vi "remove.issue.from.submap.vi"(10 "issue id":i32, 11 "map in":T1) -> (3 "map out":T1)   [LabVIEW 2024, in "manager_daemon.lvclass"]
uses:
  manager_daemon.lvclass
  type_defs/sub-map--map.ctl
  type_defs/SubData--cluster.ctl
  manager_daemon.lvclass/manager_daemon.ctl
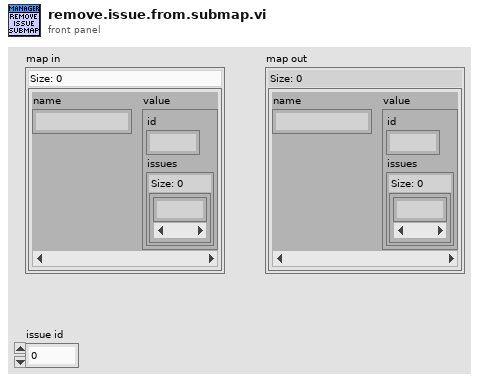
[diagram p1: front panel]
types:
  T1 = typedef "manager_daemon.lvclass/sub-map--map.ctl" = map{string, T2}
  T2 = typedef "manager_daemon.lvclass/SubData--cluster.ctl" = cluster{"id":i32, "issues":set{i32}}
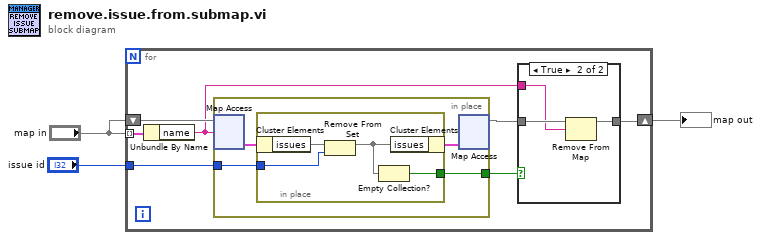
[diagram p0: block diagram]
diagram:
  n1 = for {
    tunnel: "map in" -> [w10] mode=indexing
    tunnel: "issue id" -> [w8]
    shift-right: [w5] -> w3
    shift-left: "map in" -> [w9]
    n2 = Unbundle By Name(w10) -> ("name"=w4:string)
    n3 = in-place {
      in-place-border: w8 -> [w17]
      in-place-border: [w15] -> w7
      n4 = in-place-map #1(w9, w4) -> (w18:T2)  [unwired: 1 in, 1 out]
      n5 = in-place {
        in-place-border: w17 -> [w21]
        in-place-border: [w19] -> w15
        n6 = in-place-cluster #2(w18) -> ("issues"=w22:set{i32})
        n7 = Remove From Set(10:w21, 11:w22) -> (3:w20:set{i32})  [unwired: 1 out]
        n8 = Empty Collection?(1:w20) -> (0:w19:bool)
        n9 = in-place-cluster #2("issues"=w20) -> (w16:T2)
      }
      n10 = in-place-map #1(w16) -> (w6:T1)  [unwired: 1 in, 2 out]
    }
    n11 = case shown="True" w7 {
      tunnel: w6 -> [w11 w14]
      tunnel: [w11 w13] -> w5
      tunnel: w4 -> [_ w12]
      frame False {
      }
      frame True {
        n12 = Remove From Map(10:w12, 11:w14) -> (3:w13:T1)  [unwired: 2 out]
      }
    }
  }
  "map out" <- w3
